vi "Get Tag Data.vi"(8 "error in (no error)":errorcluster, 10 "Tag ID":variant, 11 "Raw Message in":refnum<class "Raw Message.lvclass">) -> (0 "error out":errorcluster, 1 "Tag Data":variant[](array[variant]), 2 "Key not found?":bool, 3 "Raw Message out":refnum<class "Raw Message.lvclass">)   [LabVIEW 2020, in "Protobuf RAW.lvlib" / "Raw Message.lvclass"]
uses:
  Raw Message.lvclass
  Raw Message.lvclass/Raw Message.ctl
  Tag/Basic Type.lvclass
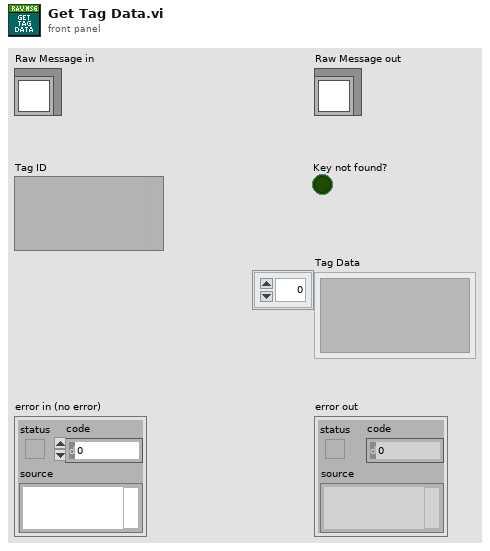
[diagram p1: front panel]
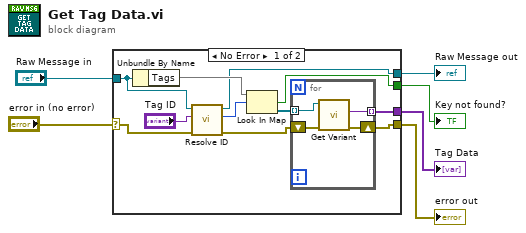
[diagram p0: block diagram]
diagram:
  n1 = case shown="No Error" "error in (no error)" {
    selector: "error in (no error)" -> [w12 w23]
    tunnel: [w17 w23] -> w5
    tunnel: [w9 w22] -> w3
    tunnel: "Raw Message in" -> [w10 w22]
    tunnel: [w13 _] -> w2
    tunnel: [w16 _] -> w1
    frame No Error {
      n2 = Unbundle By Name(w10) -> ("Tags"=w15:map{u32, refnum<class "Basic Type.lvclass">[]})
      n3 = call "Resolve ID.vi"("error in (no error)"=w12, "Tag ID / Name"="Tag ID", "Raw Message in"=w10) -> ("error out"=w11:errorcluster, "Tag ID"=w7:u32, "Raw Message out"=w9:refnum<class "Raw Message.lvclass">)  [unwired: 6 in]
      n4 = Look In Map(map=w15, key=w7) -> (key not found?=w13:bool, value=w14:refnum<class "Basic Type.lvclass">[])  [unwired: 1 in]
      n5 = for {
        tunnel: [w19] -> w16 mode=indexing
        tunnel: w14 -> [w18] mode=indexing
        shift-right: [w20] -> w17
        shift-left: w11 -> [w21]
        n6 = call-dynamic "Get Variant.vi"("error in (no error)"=w21, "Type Serializer in"=w18) -> ("error out"=w20:errorcluster, "Variant"=w19:variant)  [unwired: 7 in, 1 out]
      }
    }
    frame Error {
    }
  }
  "error out" <- w5
  "Raw Message out" <- w3
  "Key not found?" <- w2
  "Tag Data" <- w1
